vi "WPI_CANTalonSRX_SetReference.vi"(6 "Reverse Closed-Loop Output":bool, 8 "error in (no error)":errorcluster, 9 "Reverse Feedback Sensor":bool, 10 "Feedback Reference":T1, 11 "CAN Talon SRX Ref":T2={"DeviceStatus"={"status"=FALSE, "code"=0, "source"=""}, "Type"=enum."PWM", "PWM"={"PWM Channel"=enum."PWM 1", "DeadBand"={"Name"="", "maxPositivePwm"=0, "minPositivePwm"=0, "centerPwm"=0, "maxNegativePwm"=0, "minNegativePwm"=0, "angularRange"=0}}, "CAN"={"Device Number"=0, "SetOutput VI Ref"=variant(enum8{"Percent VBus", "Current", "Speed", "Position", "Voltage"} enum."Percent VBus"), "GetOutput VI Ref"=variant(refnum<k1> refnum), "Enable VI Ref"=variant(dbl 12.0), "Disable VI Ref"=variant(enum8{"Percent VBus", "Speed", "Position", "Slave", "Unchanged / Invalid", "Voltage Compensation", "Current", "Motion Profile"} enum."Percent VBus"), "Data"=variant}, "Invert"=FALSE}) -> (0 "error out":errorcluster, 3 "CAN Talon SRX Ref":T2={"DeviceStatus"={"status"=FALSE, "code"=0, "source"=""}, "Type"=enum."PWM", "PWM"={"PWM Channel"=enum."PWM 1", "DeadBand"={"Name"="", "maxPositivePwm"=0, "minPositivePwm"=0, "centerPwm"=0, "maxNegativePwm"=0, "minNegativePwm"=0, "angularRange"=0}}, "CAN"={"Device Number"=0, "SetOutput VI Ref"=variant(enum8{"Percent VBus", "Current", "Speed", "Position", "Voltage"} enum."Percent VBus"), "GetOutput VI Ref"=variant(refnum<k1> refnum), "Enable VI Ref"=variant(dbl 12.0), "Disable VI Ref"=variant(enum8{"Percent VBus", "Speed", "Position", "Slave", "Unchanged / Invalid", "Voltage Compensation", "Current", "Motion Profile"} enum."Percent VBus"), "Data"=variant}, "Invert"=FALSE})   [LabVIEW 2016]
doc: "Select the sensor used as the position process variable for the PID controller.\n\n<B>Quad Encoder</B>: Selects a quadrature encoder.\n<B>Potentiometer</B>: Selects the analog input.\n<B>None</B>: No sensor selected."
uses:
  <vilib>/Rock Robotics/WPI/MotorControl/WPI_MotorControlDeviceRef.ctl
  <vilib>/Rock Robotics/WPI/MotorControl/WPI_MotorControlType.ctl
  <vilib>/Rock Robotics/SystemInterfaces/DIO/FPGA_DIOPWMChannel.ctl
  <vilib>/Rock Robotics/WPI/PWM/WPI_PWMDeadband.ctl
  WPI_CANTalonSRX_APIFeedbackSelect.ctl
  WPI_CANTalonSRX_GlobalOps.ctl
  WPI_CANTalonSRX_FeedbackSelect.ctl
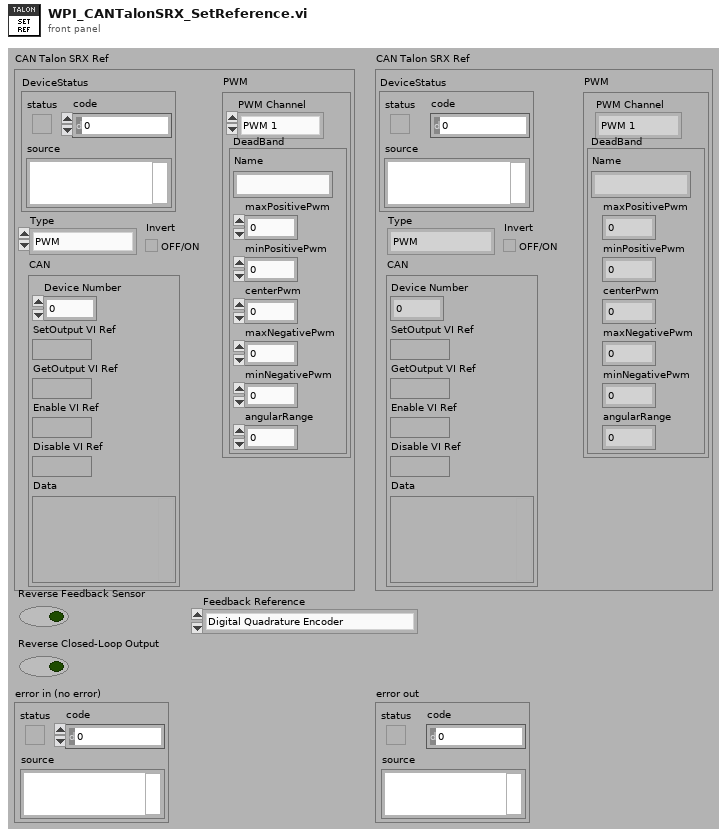
[diagram p1: front panel]
types:
  T1 = typedef "WPI_CANTalonSRX_APIFeedbackSelect.ctl" = enum16{"Digital Quadrature Encoder", "Analog Potentiometer", "Analog Encoder", "Count on Quad-A (Rising-Edge)", "Count on Quad-A (Falling-Edge)", "CTR Magnetic Enc (Absolute)", "CTR Magnetic Enc (Relative)", "Pulse Width"}
  T2 = typedef "WPI_MotorControlDeviceRef.ctl" = cluster{"DeviceStatus":errorcluster, "Type":T3, "PWM":cluster{"PWM Channel":T4, "DeadBand":T5}, "CAN":cluster{"Device Number":u8, "SetOutput VI Ref":variant, "GetOutput VI Ref":variant, "Enable VI Ref":variant, "Disable VI Ref":variant, "Data":variant}, "Invert":bool}
  T3 = typedef "WPI_MotorControlType.ctl" = enum16{"PWM", "CAN"}
  T4 = typedef "FPGA_DIOPWMChannel.ctl" = enum8{"PWM 0", "PWM 1", "PWM 2", "PWM 3", "PWM 4", "PWM 5", "PWM 6", "PWM 7", "PWM 8", "PWM 9", "PWM MXP 0", "PWM MXP 1", "PWM MXP 2", "PWM MXP 3", "PWM MXP 4", "PWM MXP 5", "PWM MXP 6", "PWM MXP 7", "PWM MXP 8", "PWM MXP 9", "Invalid"}
  T5 = typedef "WPI_PWMDeadband.ctl" = cluster{"Name":string, "maxPositivePwm":i32, "minPositivePwm":i32, "centerPwm":i32, "maxNegativePwm":i32, "minNegativePwm":i32, "angularRange":u16}
  T6 = typedef "WPI_CANTalonSRX_GlobalOps.ctl" = enum16{"Read For Send", "Write After Receive General", "Write After Receive Feedback", "Write After Receive Encoder", "Write After Receive Ain", "Write Error", "Get All", "Set Output", "Set Mode", "Set Master ID", "Set Brake Mode", "Set Reverse Feedback Sensor", "Set Reverse Closed Loop Output", "Set Override Limits", "Set Forward Limit Enabled", "Set Reverse Limit Enabled", "Set Feedback Select", "Set Profile Select", "Set Throttle Ramp Rate", "Disable", "Set Enc Codes Per Rev", "Set Num Pot Turns", "Set Control Frame Rate", "Enable Legacy Control", "Write After Receive Pulse Width", "Set Enable Frame Rate", "Write After Receive Motion Profile", "Set Motion Profile Flow Control", "Set Motion Profile Control Frame Rate", "Set Current Limit Enable"}
  T7 = typedef "WPI_CANTalonSRX_FeedbackSelect.ctl" = u8
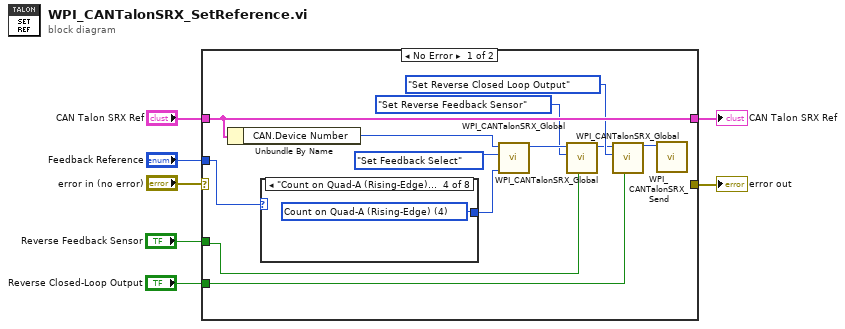
[diagram p0: block diagram]
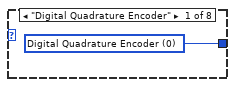
[diagram p2: hidden frame]
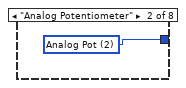
[diagram p3: hidden frame]
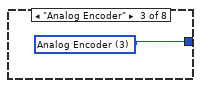
[diagram p4: hidden frame]
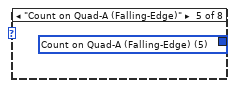
[diagram p5: hidden frame]
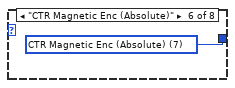
[diagram p6: hidden frame]
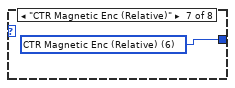
[diagram p7: hidden frame]
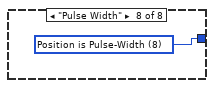
[diagram p8: hidden frame]
diagram:
  n1 = case shown="No Error" "error in (no error)" {
    selector: "error in (no error)" -> [_ w29]
    tunnel: [_ w29] -> w7
    tunnel: [w19 w28] -> w5
    tunnel: "CAN Talon SRX Ref" -> [w19 w28]
    tunnel: "Feedback Reference" -> [w16 _]
    tunnel: "Reverse Feedback Sensor" -> [w9 _]
    tunnel: "Reverse Closed-Loop Output" -> [w10 _]
    frame No Error {
      n2 = Unbundle By Name(w19) -> ("CAN.Device Number"=w18:u8)
      n3 = case shown="\"Count on Quad-A (Rising-Edge)\"" w16 {
        tunnel: [w20 w21 w22 w23 w24 w25 w26 w27] -> w15
        frame "Digital Quadrature Encoder" {
          w20 = T7 0 items=["Digital Quadrature Encoder"=0, "Analog Pot"=2, "Analog Encoder"=3, "Count on Quad-A (Rising-Edge)"=4, "Count on Quad-A (Falling-Edge)"=5, "Position is Pulse-Width"=8] ("Talon SRX Feedback Select")
        }
        frame "Analog Potentiometer" {
          w21 = T7 2 items=["Digital Quadrature Encoder"=0, "Analog Pot"=2, "Analog Encoder"=3, "Count on Quad-A (Rising-Edge)"=4, "Count on Quad-A (Falling-Edge)"=5, "Position is Pulse-Width"=8] ("Talon SRX Feedback Select")
        }
        frame "Analog Encoder" {
          w22 = T7 3 items=["Digital Quadrature Encoder"=0, "Analog Pot"=2, "Analog Encoder"=3, "Count on Quad-A (Rising-Edge)"=4, "Count on Quad-A (Falling-Edge)"=5, "Position is Pulse-Width"=8] ("Talon SRX Feedback Select")
        }
        frame "Count on Quad-A (Rising-Edge)" {
          w23 = T7 4 items=["Digital Quadrature Encoder"=0, "Analog Pot"=2, "Analog Encoder"=3, "Count on Quad-A (Rising-Edge)"=4, "Count on Quad-A (Falling-Edge)"=5, "Position is Pulse-Width"=8] ("Talon SRX Feedback Select")
        }
        frame "Count on Quad-A (Falling-Edge)" {
          w24 = T7 5 items=["Digital Quadrature Encoder"=0, "Analog Pot"=2, "Analog Encoder"=3, "Count on Quad-A (Rising-Edge)"=4, "Count on Quad-A (Falling-Edge)"=5, "Position is Pulse-Width"=8] ("Talon SRX Feedback Select")
        }
        frame "CTR Magnetic Enc (Absolute)" {
          w25 = T7 7 items=["Digital Quadrature Encoder"=0, "Analog Pot"=2, "Analog Encoder"=3, "Count on Quad-A (Rising-Edge)"=4, "Count on Quad-A (Falling-Edge)"=5, "Position is Pulse-Width"=8, "CTR Magnetic Enc (Relative)"=6, "CTR Magnetic Enc (Absolute)"=7] ("Talon SRX Feedback Select")
        }
        frame "CTR Magnetic Enc (Relative)" {
          w26 = T7 6 items=["Digital Quadrature Encoder"=0, "Analog Pot"=2, "Analog Encoder"=3, "Count on Quad-A (Rising-Edge)"=4, "Count on Quad-A (Falling-Edge)"=5, "Position is Pulse-Width"=8, "CTR Magnetic Enc (Relative)"=6, "CTR Magnetic Enc (Absolute)"=7] ("Talon SRX Feedback Select")
        }
        frame "Pulse Width" {
          w27 = T7 8 items=["Digital Quadrature Encoder"=0, "Analog Pot"=2, "Analog Encoder"=3, "Count on Quad-A (Rising-Edge)"=4, "Count on Quad-A (Falling-Edge)"=5, "Position is Pulse-Width"=8] ("Talon SRX Feedback Select")
        }
      }
      n4 = call "WPI_CANTalonSRX_Global.vi"("Set Number"=w15, "Operation"=WPI_CANTalonSRX_GlobalOps."Set Feedback Select", "Device ID (0)"=w18) -> ("Device ID Out"=w14:u8)  [unwired: 6 in, 2 out]
      n5 = call "WPI_CANTalonSRX_Global.vi"("Set Boolean"=w9, "Operation"=WPI_CANTalonSRX_GlobalOps."Set Reverse Feedback Sensor", "Device ID (0)"=w14) -> ("Device ID Out"=w11:u8)  [unwired: 6 in, 2 out]
      n6 = call "WPI_CANTalonSRX_Global.vi"("Set Boolean"=w10, "Operation"=WPI_CANTalonSRX_GlobalOps."Set Reverse Closed Loop Output", "Device ID (0)"=w11) -> ("Device ID Out"=w8:u8)  [unwired: 6 in, 2 out]
      n7 = call "WPI_CANTalonSRX_Send.vi"("Device ID (0)"=w8) -> ()  [unwired: 10 in, 1 out]
    }
    frame Error {
    }
  }
  "CAN Talon SRX Ref" <- w5
  "error out" <- w7
